vi "Download Complete.vi"(7 "MulticolumnListbox in":refnum<vi>, 8 "Error In":errorcluster, 11 "Dependency Config":T1) -> (0 "Error Out":errorcluster, 3 "Dependency Config":T1)   [LabVIEW 2014, in "LMH-Toolbox.lvlib" / "LMH-Installer Tools.lvlib"]
uses:
  <vilib>/MakerHub/Toolbox/Private/Installer Tools/LMH-Installer Tools.lvlib
  <vilib>/MakerHub/Toolbox/Private/Installer Tools/Private/Type Defs/Dependency Config.ctl
  <vilib>/MakerHub/Toolbox/Private/Installer Tools/Private/Type Defs/Dependecy.ctl
  <vilib>/MakerHub/Toolbox/Private/Web/Type Defs/Download Task.ctl
  <vilib>/MakerHub/Toolbox/Private/Web/LMH-Web.lvlib
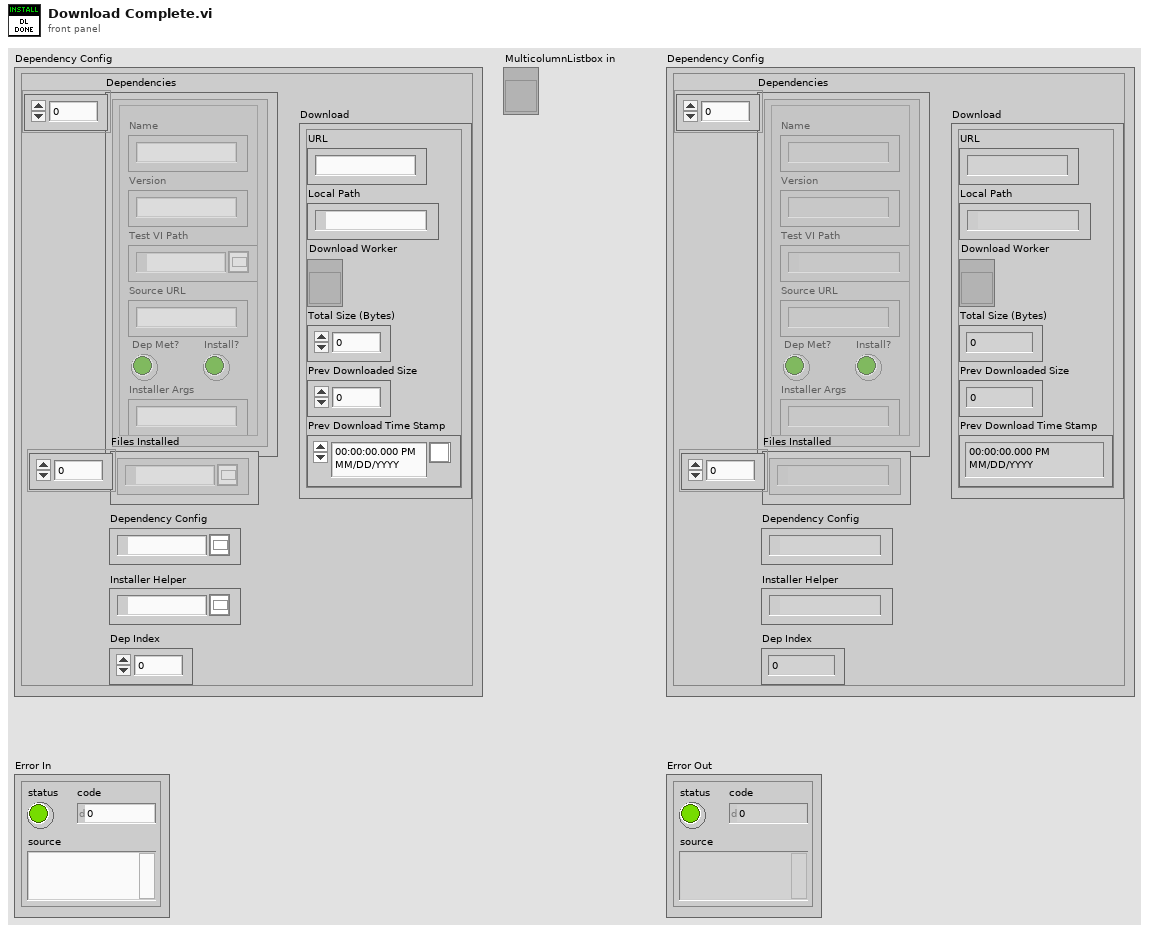
[diagram p1: front panel]
types:
  T1 = typedef "LMH-Toolbox.lvlib/LMH-Installer Tools.lvlib/Dependency Config.ctl" = cluster{"Dependencies":T2[], "Files Installed":path[], "Dependency Config":path, "Installer Helper":path, "Dep Index":i32, "Download":T3}
  T2 = typedef "LMH-Toolbox.lvlib/LMH-Installer Tools.lvlib/Dependecy.ctl" = cluster{"Name":string, "Version":string, "Test VI Path":path, "Source URL":string, "Dep Met?":bool, "Install?":bool, "Installer Args":string}
  T3 = typedef "LMH-Toolbox.lvlib/LMH-Web.lvlib/Download Task.ctl" = cluster{"URL":string, "Local Path":path, "Download Worker":refnum<vi>, "Total Size (Bytes)":u64, "Prev Downloaded Size":u64, "Prev Download Time Stamp":timestamp}
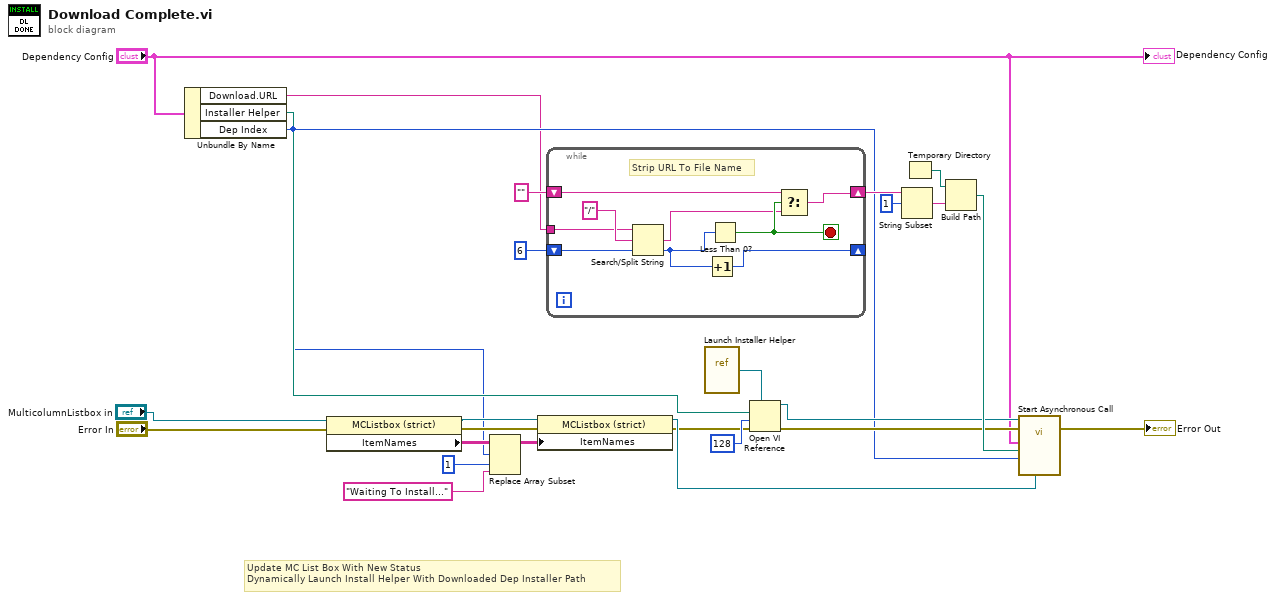
[diagram p0: block diagram]
diagram:
  # "Update MC List Box With New Status\nDynamically Launch Install Helper With Downloaded Dep Installer Path"
  n1 = Unbundle By Name("Dependency Config") -> ("Download.URL"=w1:string, "Installer Helper"=w3:path, "Dep Index"=w2:i32)
  n2 = property on="Property Node" class="MCListbox (strict)"(reference="MulticolumnListbox in", error in="Error In") -> (reference out=w7:refnum<vi>, error out=w23:errorcluster, "ItemNames"=w20:string[][])
  n3 = Replace Array Subset(array=w20, new element="Waiting To Install..." ("new element/subarray"), index (row)=w2, index (col)=1 ("disabled index (col)")) -> (w24:string[][])
  n4 = property on="Property Node" class="MCListbox (strict)"(reference=w7, error in=w23, "ItemNames"=w24) -> (reference out=w8:refnum<vi>, error out=w6:errorcluster)
  n5 = while {
    shift-right: [w32] -> _
    shift-left: 6 ("offset (0)") -> [w34]
    shift-right: [w29] -> w11
    shift-left: "" ("search string/char (-)") -> [w30]
    tunnel: w1 -> [w27]
    stop <- w31 stop-if-true
    # "Strip URL To File Name"
    n6 = Search/Split String(string=w27, search string/char (-)="/", offset (0)=w34) -> (match + rest of string=w28:string, offset of match=w33:i32)  [unwired: 1 out]
    n7 = Increment(x=w33) -> (x+1=w32:i32)
    n8 = Less Than 0?(x=w33) -> (x < 0?=w31:bool)
    n9 = Select(t=w30, s=w31, f=w28) -> (s? t:f=w29:string)
  }
  n10 = vi-ref <vilib>:"Launch Installer Helper.vi"() -> (w17:refnum<vi>)
  n11 = Open VI Reference(type specifier VI Refnum (for type only)=w17, vi path=w3, options=128, error in (no error)=w6) -> (vi reference=w18:refnum<vi>, error out=w5:errorcluster)  [unwired: 2 in]
  n12 = String Subset(string=w11, offset (0)=1) -> (substring=w14:string)  [unwired: 1 in]
  n13 = Temporary Directory() -> (w15:path)
  n14 = Build Path(base path=w15, name or relative path=w14) -> (appended path=w26:path)
  n15 = call-by-ref "Start Asynchronous Call"(reference=w18, error in=w5, "Listbox Ref"=w8, "Dep Index"=w2, "File Path Control"=w26, "Dependecy Config"="Dependency Config") -> (error out=→"Error Out":errorcluster)  [unwired: 7 in, 2 out]
  "Dependency Config" <- "Dependency Config"
